vi "DailyReport.vi"() -> ()   [LabVIEW 2012]
panel:
  out "Boolean":bool
  in  "From Date (起日)":string="2014/9/20"
  in  "離開":bool
  in  "執行":bool
  in  "Shift (班別)":string(combo)
  in  "End Date (ùら)":string="2014/9/24"
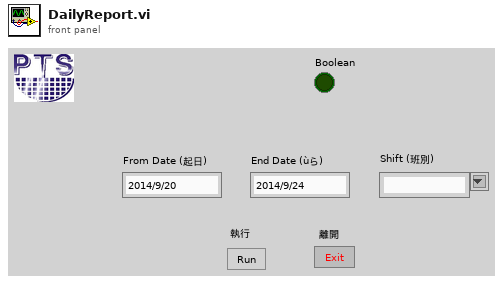
[diagram p1: front panel]
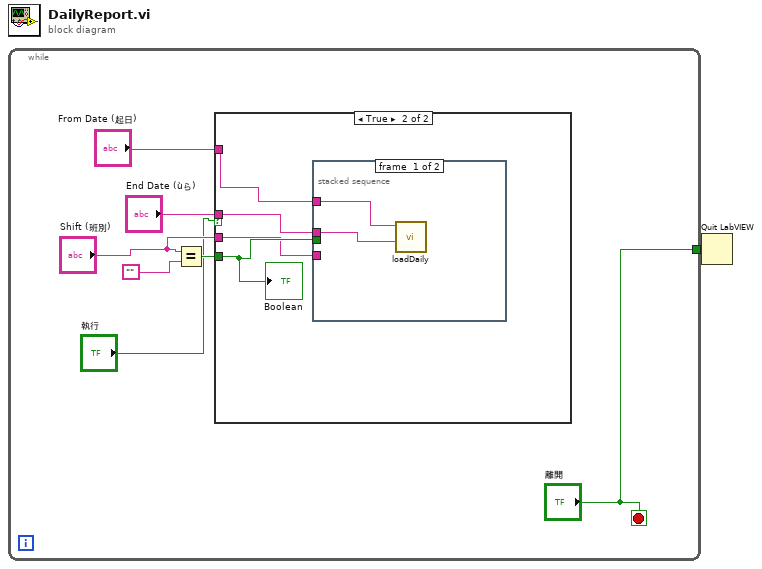
[diagram p0: block diagram]
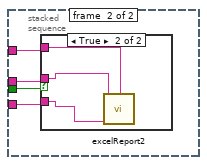
[diagram p3: hidden frame]
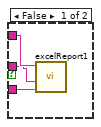
[diagram p4: hidden frame]
diagram:
  n1 = while {
    tunnel: ["離開"] -> w1
    stop <- "離開" stop-if-true
    n2 = Equal?(x="Shift (班別)", y="") -> (x = y?=w7:bool)
    n3 = case shown="True" "執行" {
      tunnel: "From Date (起日)" -> [_ w12]
      tunnel: w7 -> [_ w11]
      tunnel: "End Date (ùら)" -> [_ w10]
      tunnel: "Shift (班別)" -> [_ w9]
      frame False {
      }
      frame True {
        n4 = stacked-sequence {
          tunnel: w12 -> [w14 w18]
          tunnel: w11 -> [_ w16]
          tunnel: w10 -> [w13 w17]
          tunnel: w9 -> [_ w15]
          frame #0 {
            n5 = call "loadDaily.vi"("end date"=w13, "begin date"=w14) -> ()  [unwired: 9 in, 1 out]
          }
          frame #1 {
            n6 = case shown="True" w16 {
              tunnel: w18 -> [w21 w24]
              tunnel: w17 -> [w20 w23]
              tunnel: w15 -> [w19 w22]
              frame False {
                n7 = call "excelReport1.vi"("Shift"=w19, "End Date"=w20, "From Date"=w21) -> ()  [unwired: 9 in]
              }
              frame True {
                n8 = call "excelReport2.vi"("Shift"=w22, "End Date"=w23, "From Date"=w24) -> ()  [unwired: 9 in]
              }
            }
          }
        }
        "Boolean" <- w11
      }
    }
  }
  n9 = Quit LabVIEW(quit? (T)=w1) -> ()
